vi "Get Rx Monitor Size Distribution.vi"() -> (3 "Channel Array":string[](array[string]))   [LabVIEW 2020, in "AIM ARINC 664 GUID Utility.lvlib"]
uses:
  AIM ARINC 664 GUID Utility.lvlib
  Scripting/Constants.vi
  Scripting/AIM ARINC 664 Scripting.lvlib
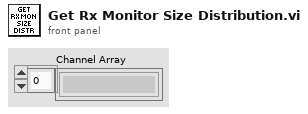
[diagram p1: front panel]
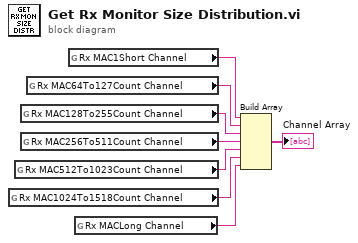
[diagram p0: block diagram]
diagram:
  n1 = global read "Constants.vi" "Rx MAC1024To1518Count Channel"() -> (w3:string)
  n2 = global read "Constants.vi" "Rx MAC512To1023Count Channel"() -> (w4:string)
  n3 = global read "Constants.vi" "Rx MAC128To255Count Channel"() -> (w6:string)
  n4 = global read "Constants.vi" "Rx MAC256To511Count Channel"() -> (w5:string)
  n5 = global read "Constants.vi" "Rx MAC64To127Count Channel"() -> (w7:string)
  n6 = global read "Constants.vi" "Rx MAC1Short Channel"() -> (w8:string)
  n7 = global read "Constants.vi" "Rx MACLong Channel"() -> (w2:string)
  n8 = Build Array(w8, w7, w6, w5, w4, w3, w2) -> (→"Channel Array":string[])
